vi "全局_综合生物毒性.vi"() -> ()   [LabVIEW 2016, in "综合生物毒性.lvlib"]
uses:
  <vilib>/Plasmionique/MB Master/MB_Master_Serial/MB_Master_Serial.lvclass
panel:
  out "启动时间":timestamp
  in  "测量模式":string
  out "纯水时间":timestamp
  out "质控时间":timestamp
  out "水样时间":timestamp
  out "系统时间":timestamp
  out "数据时间":timestamp
  out "MB_Serial session":refnum<class "MB_Master_Serial.lvclass">
  in  "VISA Resource":refnum<visa-resource-name>
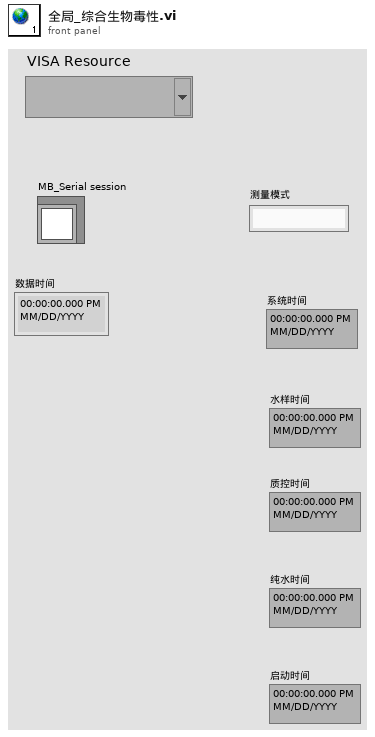
[diagram p1: front panel]
diagram:
